vi "60percent.vi"(11 "In":dbl) -> (3 "Out":dbl)   [LabVIEW 2020]
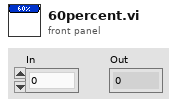
[diagram p1: front panel]
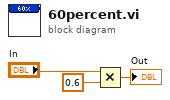
[diagram p0: block diagram]
diagram:
  n1 = Multiply(x="In", y=0.6) -> (x*y=→"Out":dbl)
